vi "robotOrientatedToBall.vi"(8 "error in (no error)":errorcluster, 9 "Robot":refnum<class "Robot.lvclass">, 10 "Game":refnum<class "Game.lvclass">, 11 "Utilities in":refnum<class "Utilities.lvclass">) -> (0 "error out":errorcluster, 2 "Orientation":dbl, 3 "Utilities out":refnum<class "Utilities.lvclass">)   [LabVIEW 2018, in "Utilities.lvclass"]
uses:
  Utilities.lvclass
  Game_class/Game.lvclass
  Robot_class/Robot.lvclass
  C:/Users/Ronaldo/Desktop/Phoenix/SSL_AI/Object_class/Object.lvclass
  Game_class/Game.lvclass/Game.ctl
  Object_class/Object.lvclass/Object.ctl
  Object_class/Read x.vi
  Object_class/Read y.vi
  Game_class/Read BallRef.vi
  Ball_class/Ball.lvclass
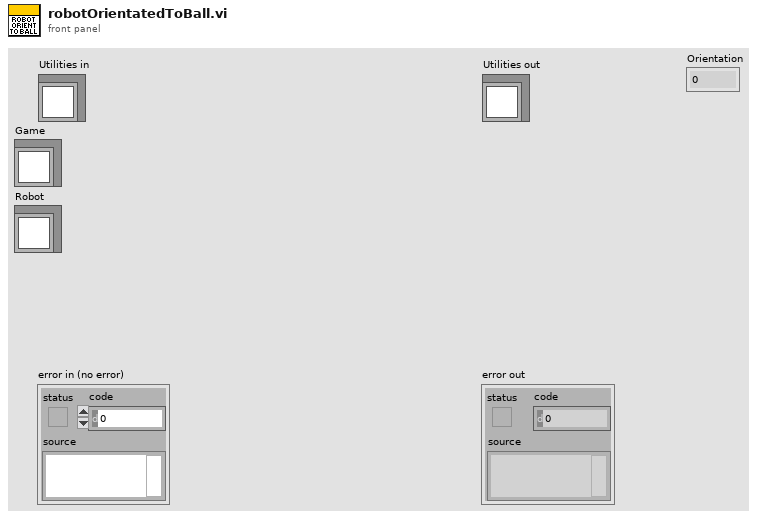
[diagram p1: front panel]
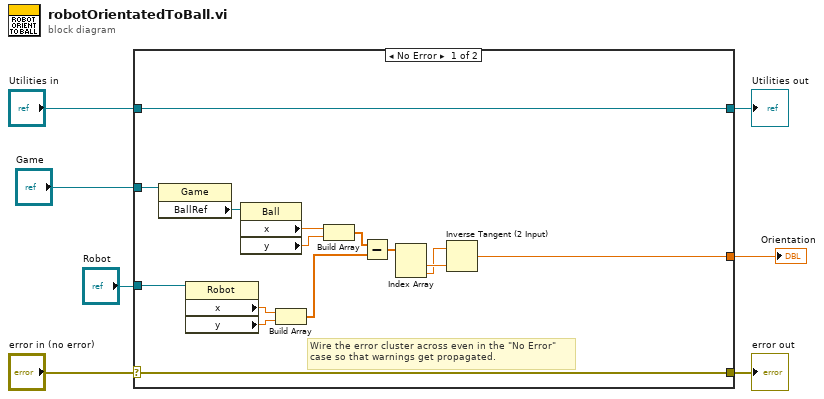
[diagram p0: block diagram]
diagram:
  n1 = case shown="No Error" "error in (no error)" {
    selector: "error in (no error)" -> [w21 w24]
    tunnel: [w21 w24] -> w6
    tunnel: [w22 w23] -> w4
    tunnel: "Utilities in" -> [w22 w23]
    tunnel: "Game" -> [w20 _]
    tunnel: "Robot" -> [w15 _]
    tunnel: [w8 _] -> w1
    frame No Error {
      # "Wire the error cluster across even in the \"No Error\"\ncase so that warnings get propagated."
      n2 = property class="Game"(reference=w20) -> ("BallRef"=w19:refnum<class "Ball.lvclass">)  [unwired: 1 in, 2 out]
      n3 = property class="Robot"(reference=w15) -> ("x"=w14:dbl, "y"=w13:dbl)  [unwired: 1 in, 2 out]
      n4 = property class="Ball"(reference=w19) -> ("x"=w18:dbl, "y"=w17:dbl)  [unwired: 1 in, 2 out]
      n5 = Build Array(w14, w13) -> (w12:dbl[])
      n6 = Build Array(w18, w17) -> (w16:dbl[])
      n7 = Subtract(x=w16, y=w12) -> (x-y=w11:dbl[])
      n8 = Index Array(array=w11) -> (element #1=w10:dbl, element #2=w9:dbl)  [unwired: 2 in]
      n9 = Inverse Tangent (2 Input)(1:w10, 2:w9) -> (0:w8:dbl)
    }
    frame Error {
    }
  }
  "error out" <- w6
  "Utilities out" <- w4
  "Orientation" <- w1
